vi "List Parts.vi"(7 "Request parameters":T5={"Max parts"=-1, "Part number marker"=1} {"Part number marker" min=1 max=10000; "Max parts" max=1000}, 8 "error in (no error)":errorcluster, 9 "Bucket":string, 10 "Path":string, 11 "Upload ID":string) -> (0 "error out":errorcluster, 3 "ListPartsResult":T1 {"Parts"."PartNumber" min=1 max=10000})   [LabVIEW 2011, in "LV Interface for Amazon S3.lvlib"]
doc: "This operation <B>lists the parts that have been uploaded</B> for a specific multipart upload. This operation <B>must include the upload ID</B>, which you obtain <B>by calling Get Multipart Upload ID.vi</B>."
uses:
  LV Interface for Amazon S3.lvlib
  Typedefs/AMZ_S3_API_List Parts Request Parameters.ctl
  Typedefs/AMZ_S3_API_ListPartsResult.ctl
  Typedefs/AMZ_S3_API_Owner.ctl
  Typedefs/AMZ_S3_Storage Class.ctl
  Typedefs/AMZ_S3_Multipart Upload Part Data.ctl
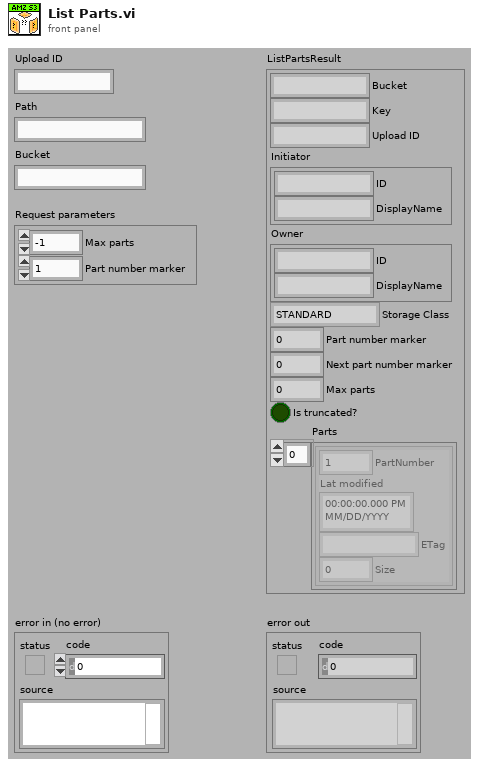
[diagram p1: front panel]
types:
  T1 = typedef "LV Interface for Amazon S3.lvlib/AMZ_S3_API_ListPartsResult.ctl" = cluster{"Bucket":string, "Key":string, "Upload ID":string, "Initiator":T2, "Owner":T2, "Storage Class":T3, "Part number marker":u16, "Next part number marker":u16, "Max parts":u16, "Is truncated?":bool, "Parts":T4[]}
  T2 = typedef "LV Interface for Amazon S3.lvlib/AMZ_S3_API_Owner.ctl" = cluster{"ID":string, "DisplayName":string}
  T3 = typedef "LV Interface for Amazon S3.lvlib/AMZ_S3_Storage Class.ctl" = enum16{"STANDARD", "REDUCED_REDUNDANCY"}
  T4 = typedef "LV Interface for Amazon S3.lvlib/AMZ_S3_Multipart Upload Part Data.ctl" = cluster{"PartNumber":u16, "Lat modified":timestamp, "ETag":string, "Size":u64}
  T5 = typedef "LV Interface for Amazon S3.lvlib/AMZ_S3_API_List Parts Request Parameters.ctl" = cluster{"Max parts":i16, "Part number marker":u16}
  T6 = typedef "LV Interface for Amazon S3.lvlib/AMZ_S3_Call Results.ctl" = enum16{"Success", "UndefinedError", "AccessDenied", "AccountProblem", "AmbiguousGrantByEmailAddress", "BadDigest", "BucketAlreadyExists", "BucketAlreadyOwnedByYou", "BucketNotEmpty", "CredentialsNotSupported", "CrossLocationLoggingProhibited", "EntityTooSmall", "EntityTooLarge", "ExpiredToken", "IllegalVersioningConfigurationException", "IncompleteBody", "IncorrectNumberOfFilesInPostRequest", "InlineDataTooLarge", "InternalError", "InvalidAccessKeyId", "InvalidAddressingHeader", "InvalidArgument", "InvalidBucketName", "InvalidDigest", "InvalidLocationConstraint", "InvalidPart", "InvalidPartOrder", "InvalidPayer", "InvalidPolicyDocument", "InvalidRange", "InvalidSecurity", "InvalidSOAPRequest", "InvalidStorageClass", "InvalidTargetBucketForLogging", "InvalidToken", "InvalidURI", "KeyTooLong", "MalformedACLError", "MalformedPOSTRequest", "MalformedXML", "MaxMessageLengthExceeded", "MaxPostPreDataLengthExceededError", "MetadataTooLarge", "MethodNotAllowed", "MissingAttachment", "MissingContentLength", "MissingRequestBodyError", "MissingSecurityElement", "MissingSecurityHeader", "NoLoggingStatusForKey", "NoSuchBucket", "NoSuchKey", "NoSuchUpload", "NoSuchVersion", "NotImplemented", "NotSignedUp", "OperationAborted", "PermanentRedirect", "PreconditionFailed", "Redirect", "RequestIsNotMultiPartContent", "RequestTimeout", "RequestTimeTooSkewed", "RequestTorrentOfBucketError", "SignatureDoesNotMatch", "SlowDown", "TemporaryRedirect", "TokenRefreshRequired", "TooManyBuckets", "UnexpectedContent", "UnresolvableGrantByEmailAddress", "UserKeyMustBeSpecified", "LabVIEWError"}
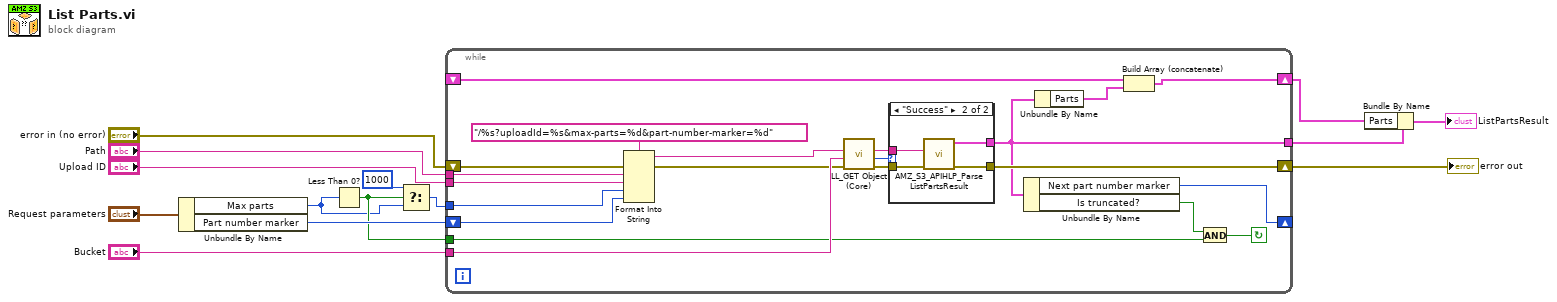
[diagram p0: block diagram]
diagram:
  n1 = Unbundle By Name("Request parameters") -> ("Max parts"=w6:i16, "Part number marker"=w11:u16)
  n2 = Less Than 0?(x=w6) -> (x < 0?=w7:bool)
  n3 = Select(t=i16 1000, s=w7, f=w6) -> (s? t:f=w5:i16)
  n4 = while {
    tunnel: "Path" -> [w35]
    tunnel: "Upload ID" -> [w34]
    tunnel: "Bucket" -> [w31]
    tunnel: [w19] -> w3
    shift-right: [w30] -> w8
    shift-left: "error in (no error)" -> [w32]
    shift-right: [w15] -> _
    shift-left: w11 -> [w33]
    tunnel: w7 -> [w21]
    tunnel: w5 -> [w23]
    shift-right: [w17] -> w1
    shift-left: _ -> [w16]
    stop <- w20 continue-if-true
    n5 = Format Into String(format string="/%s?uploadId=%s&max-parts=%d&part-number-marker=%d", error in=w32, w35, w34, w23, w33) -> (resulting string=w27:string, error out=w28:errorcluster)  [unwired: 1 in]
    n6 = call "LL_GET Object (Core).vi"("error in (no error)"=w28, "Bucket"=w31, "Path and query string"=w27) -> ("error out"=w25:errorcluster, "Call Result"=w26:T6, "Response body"=w24:string)  [unwired: 5 in, 1 out]
    n7 = case shown="\"Success\"" w26 {
      tunnel: w25 -> [w36 w40]
      tunnel: w24 -> [_ w39]
      tunnel: [_ w38] -> w19
      tunnel: [w36 w37] -> w30
      frame Default {
      }
      frame "Success" {
        n8 = call "AMZ_S3_APIHLP_Parse ListPartsResult.vi"("error in (no error)"=w40, "Response body"=w39) -> ("error out"=w37:errorcluster, "ListPartsResult"=w38:T1)  [unwired: 8 in]
      }
    }
    n9 = Unbundle By Name(w19) -> ("Next part number marker"=w15:u16, "Is truncated?"=w22:bool)
    n10 = Unbundle By Name(w19) -> ("Parts"=w18:T4[])
    n11 = Build Array (concatenate)(w16, w18) -> (w17:T4[])
    n12 = And(x=w22, y=w21) -> (x .and. y?=w20:bool)
  }
  "error out" <- w8
  n13 = Bundle By Name(cluster=w3, "Parts"=w1) -> (→"ListPartsResult":T1)
